vi "ReadCamera.vi"() -> ()   [LabVIEW 2021]
panel:
  out "Barcode Grading Report (Barcode Reader 1)":T1(array[cluster])
  out "Complete Data (Barcode Reader 1)":string[](array[string])
  out "Barcodes (Barcode Reader 1)":T2(array[cluster]) {"Confidence Level" format="%.2f"; "Barcode Type" items=["Reserved", "Codabar", "Code 39", "Code 93", "Code 128", "EAN 8", "EAN 13", "Interleaved 2 of 5", "MSI", "UPCA", "Pharmacode", "RSS Limited"]; "Bounding Box"."y" format="%.2f"; "Bounding Box"."x" format="%.2f"}
  in  "OK Button":bool
  out "Image":T3(plugin-control)
  in  "stop":bool
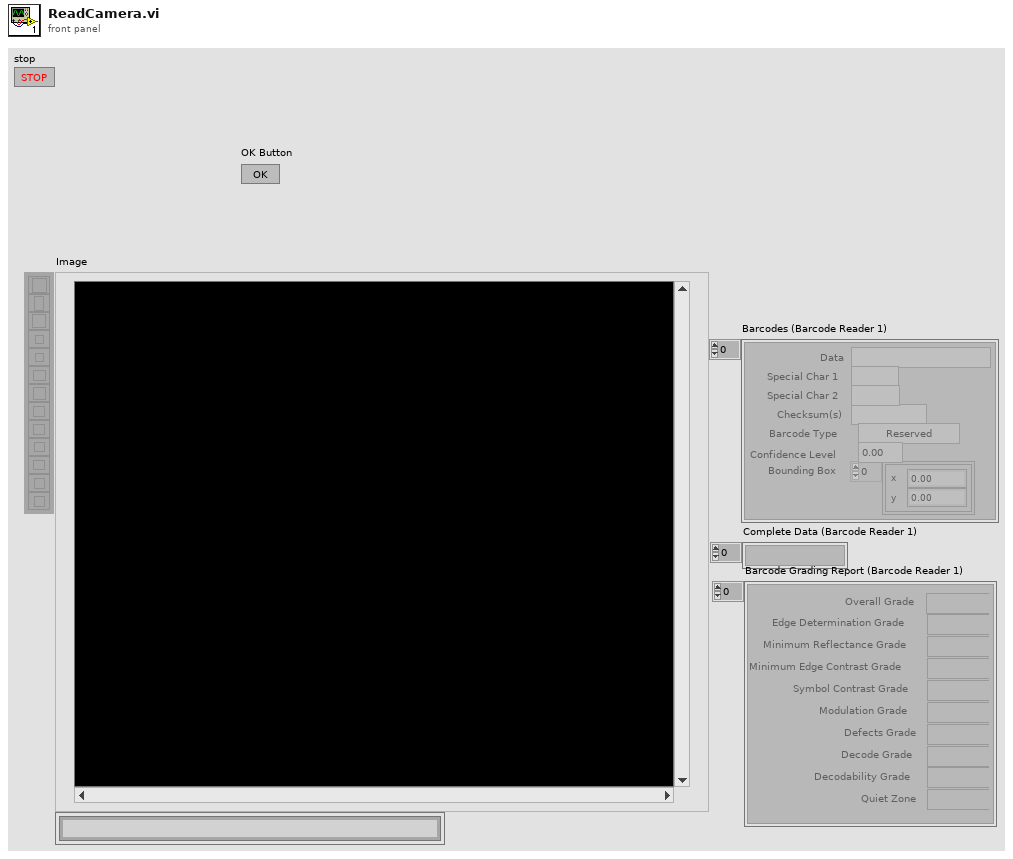
[diagram p1: front panel]
types:
  T1 = cluster{"Overall Grade":string, "Edge Determination Grade":string, "Minimum Reflectance Grade":string, "Minimum Edge Contrast Grade":string, "Symbol Contrast Grade":string, "Modulation Grade":string, "Defects Grade":string, "Decode Grade":string, "Decodability Grade":string, "Quiet Zone":string}[]
  T2 = cluster{"Data":string, "Special Char 1":string, "Special Char 2":string, "Checksum(s)":string, "Barcode Type":u32, "Confidence Level":sgl, "Bounding Box":cluster{"x":sgl, "y":sgl}[]}[]
  T3 = typedef "IMAQ Image.ctl" = refnum<image>
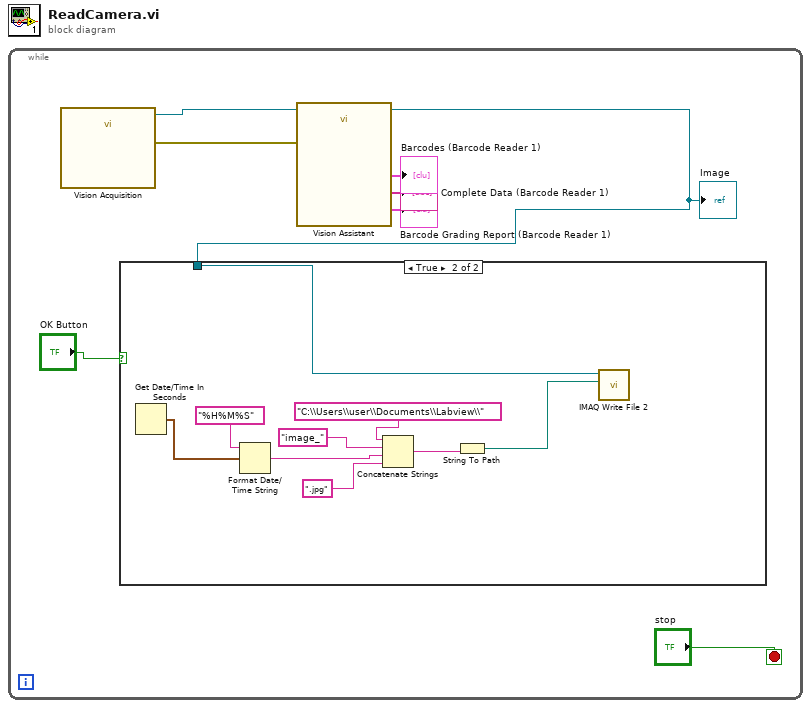
[diagram p0: block diagram]
diagram:
  n1 = while {
    stop <- "stop" stop-if-true
    n2 = call "Vision Acquisition"() -> ("Image Out"=w8:T3, "error out"=w7:errorcluster)  [unwired: 25 in, 1 out]
    n3 = call "Vision Assistant"("Image In"=w8, "error in"=w7) -> ("Image Out"=w5:T3, "Barcodes (Barcode Reader 1)"=→"Barcodes (Barcode Reader 1)":T2, "Complete Data (Barcode Reader 1)"=→"Complete Data (Barcode Reader 1)":string[], "Barcode Grading Report (Barcode Reader 1)"=→"Barcode Grading Report (Barcode Reader 1)":T1)  [unwired: 21 in, 1 out]
    "Image" <- w5
    n4 = case shown="True" "OK Button" {
      tunnel: w5 -> [_ w17]
      frame False {
      }
      frame True {
        n5 = Get Date/Time In Seconds() -> (seconds since 1Jan1904=w16:timestamp)
        n6 = Format Date/Time String(time format string (%c)="%H%M%S", seconds (now)=w16) -> (date/time string=w13:string)  [unwired: 1 in]
        n7 = Concatenate Strings("C:\\Users\\user\\Documents\\Labview\\" ("string"), "image_" ("string"), w13, ".jpg" ("string")) -> (w10:string)
        n8 = String To Path(string=w10) -> (path=w9:path)
        n9 = call-poly "IMAQ Write File 2"("File Path"=w9, "Image"=w17) -> ()  [unwired: 8 in, 2 out]
      }
    }
  }
